vi "AudioTest.Calibrate Generated Waveform, Lookup Amplitude based on Frequency.vi"(10 "Waveform Cal":cluster{"Freq":dbl[], "Gain":dbl[]}, 11 "Freq":dbl) -> (3 "Gain":dbl)   [LabVIEW 2018]
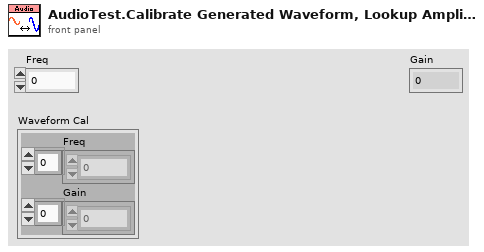
[diagram p1: front panel]
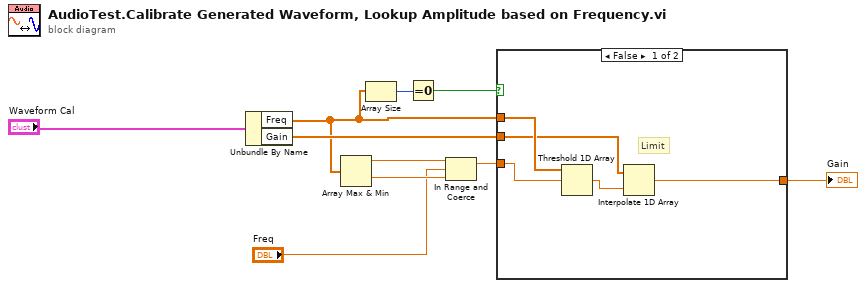
[diagram p0: block diagram]
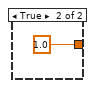
[diagram p2: hidden frame]
diagram:
  n1 = Unbundle By Name("Waveform Cal") -> ("Freq"=w3:dbl[], "Gain"=w7:dbl[])
  n2 = Array Max & Min(array=w3) -> (max value=w9:dbl, min value=w8:dbl)  [unwired: 2 out]
  n3 = Array Size(array=w3) -> (size(s)=w2:i32)
  n4 = Equal To 0?(x=w2) -> (x = 0?=w1:bool)
  n5 = In Range and Coerce(upper limit=w9, x="Freq", lower limit=w8) -> (coerced(x)=w4:dbl)  [unwired: 1 out]
  n6 = case shown="False" w1 {
    tunnel: w3 -> [w15 _]
    tunnel: w7 -> [w13 _]
    tunnel: [w12 1.0] -> w5
    tunnel: w4 -> [w11 _]
    frame False {
      # "Limit"
      n7 = Threshold 1D Array(2:w11, 3:w15) -> (0:w14:dbl)  [unwired: 1 in]
      n8 = Interpolate 1D Array(1:w14, 2:w13) -> (0:w12:dbl)
    }
    frame True {
    }
  }
  "Gain" <- w5
